vi "LokaleHysteresenBerechnung.vi"(8 "error in":errorcluster, 11 "TempKurve":dbl[](array[numeric])) -> (0 "error out":errorcluster, 3 "lokale Hysterese":dbl)   [LabVIEW 2024]
panel:
  in  "lokales Min":dbl
  in  "lokales Max":dbl
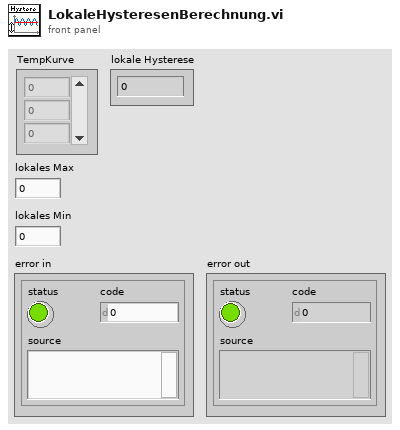
[diagram p1: front panel]
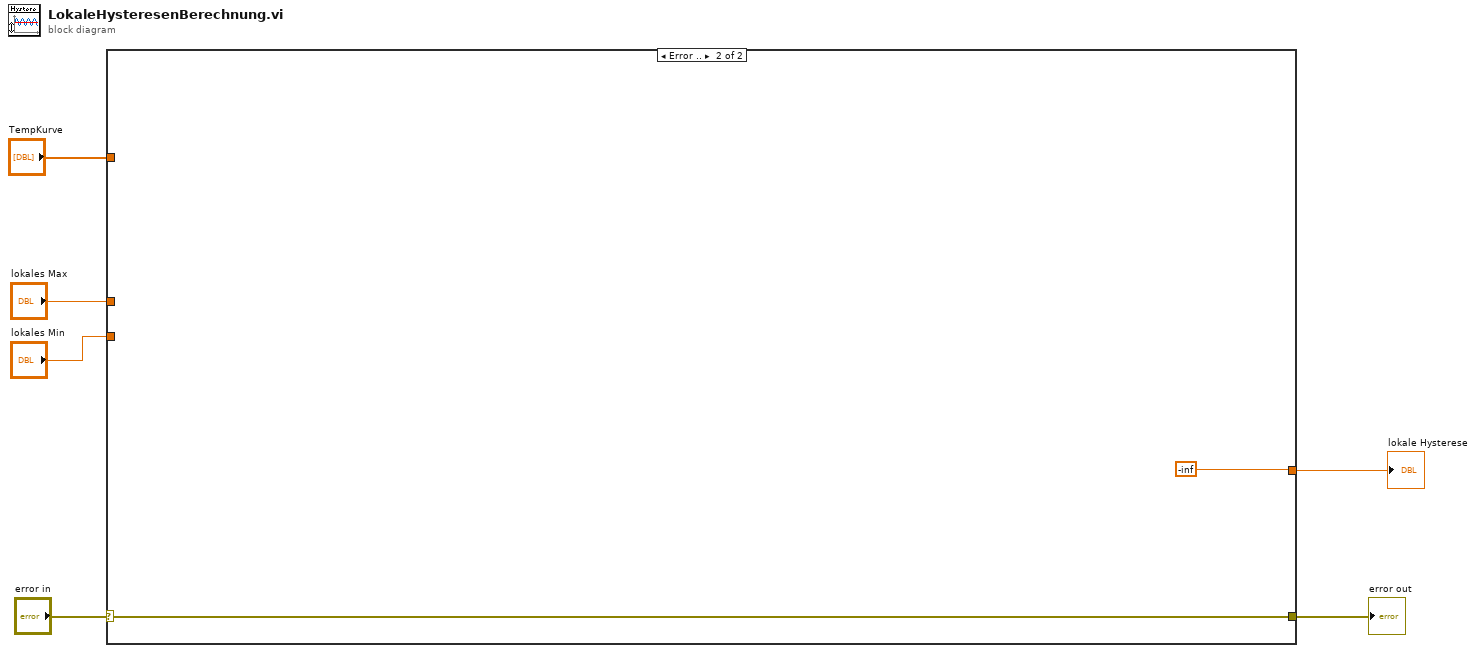
[diagram p0: block diagram]
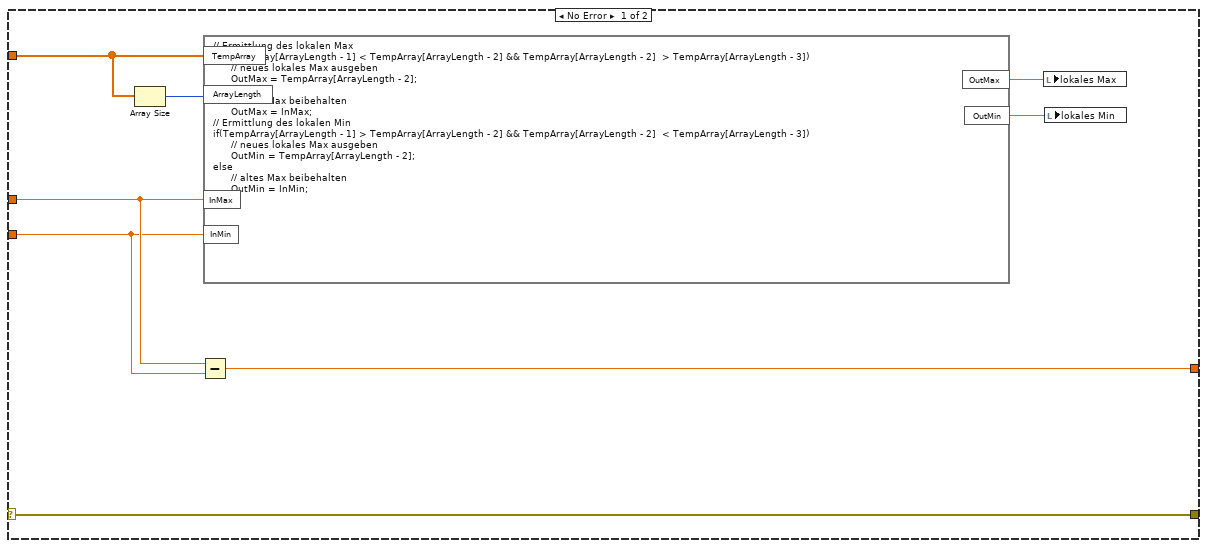
[diagram p2: hidden frame]
diagram:
  n1 = case shown="Error .." "error in" {
    selector: "error in" -> [w14 w16]
    tunnel: [w14 w16] -> w5
    tunnel: "TempKurve" -> [w12 _]
    tunnel: "lokales Max" -> [w9 _]
    tunnel: "lokales Min" -> [w8 _]
    tunnel: [w7 -inf] -> w1
    frame No Error {
      n2 = Array Size(array=w12) -> (size(s)=w13:i32)
      n3 = Subtract(x=w9, y=w8) -> (x-y=w7:dbl)
      n4 = formula code="// Ermittlung des lokalen Max\nif(TempArray[ArrayLength - 1] < TempArray[ArrayLength - 2] && TempArray[ArrayLength - 2]  > TempArray[ArrayLength - 3])\n      // neues lokales Max ausgeben\n      OutMax = TempArray[ArrayLength - 2];\nelse\n      // altes Max beibehalten\n      OutMax = InMax;\n// Ermittlung des lokalen Min\nif(TempArray[ArrayLength - 1] > TempArray[ArrayLength - 2] && TempArray[ArrayLength - 2]  < TempArray[ArrayLength - 3])\n      // neues lokales Max ausgeben\n      OutMin = TempArray[ArrayLength - 2];\nelse\n      // altes Max beibehalten\n      OutMin = InMin;"("TempArray"=w12, "ArrayLength"=w13, "InMax"=w9, "InMin"=w8) -> ("OutMax"=w11:dbl, "OutMin"=w10:dbl)
      n5 = local write "lokales Max"(w11) -> ()
      n6 = local write "lokales Min"(w10) -> ()
    }
    frame Error {
    }
  }
  "lokale Hysterese" <- w1
  "error out" <- w5
